vi "getControlData_singleAxis_linear.vi"(11 "system matricec path":path=path "C:/Users/arnold/Documents/MATLAB/AFM_MPC/data/exp_multiAxis.csv") -> (2 "AllMatrix":dbl[](array[numeric]), 3 "ControlParamsMpc":T1={"umax"=3.0, "NS"=0, "ref_f_VEC"=[0.0, 0.0], "Nu11_22"=[0.0, 0.0], "u0"=[0.0, 0.0]})   [LabVIEW 2017]
uses:
  fpga_VIs/fixed-point/typeDefs/FXPControlParams_distEst.ctl
  <vilib>/Utility/file.llb/Read From Spreadsheet File (DBL).vi
panel:
  # "This vi gets control data from a .csv file. It expects the data in\nthe following format:\n| B,   Ki       |\n| L,    Nbar |\n|K',   Ns      |\n|C',   Nd     |\n|Arn,  ref    |\n|.         0      |\n|.         0      |"
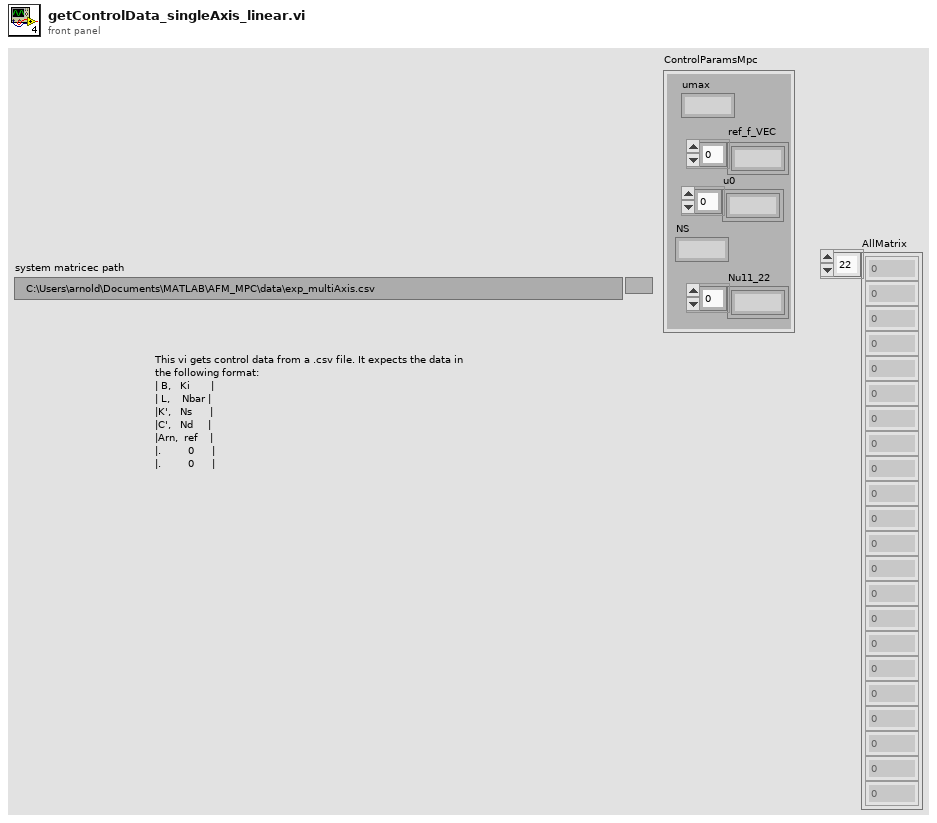
[diagram p1: front panel]
types:
  T1 = typedef "FXPControlParams_distEst.ctl" = cluster{"umax":fxp<+/-,18,5>, "NS":u8, "ref_f_VEC":fxp<+/-,32,5>[], "Nu11_22":fxp<+/-,32,5>[], "u0":fxp<+/-,32,5>[]}
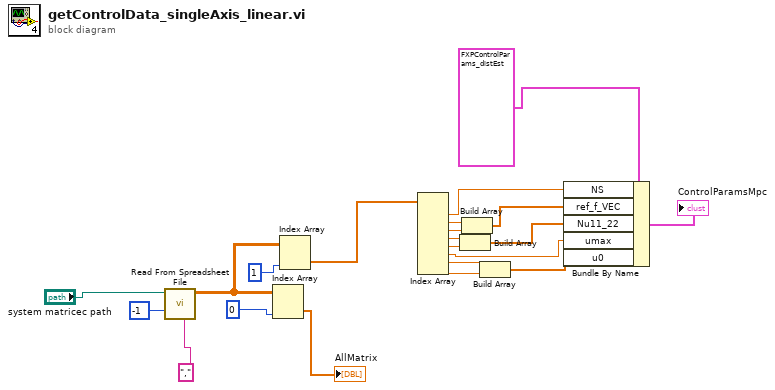
[diagram p0: block diagram]
diagram:
  n1 = call-poly <vilib>:"Read From Spreadsheet File.vi"("delimiter (\\t)"=",", "number of rows (all:-1)"=-1, "file path (dialog if empty)"="system matricec path") -> ("all rows"=w16:dbl[][])  [unwired: 4 in, 4 out]
  n2 = Index Array(array=w16, index (col)=0 ("dimension size")) -> (element=→"AllMatrix":dbl[])  [unwired: 1 in]
  n3 = Index Array(array=w16, index (col)=1 ("dimension size")) -> (element=w19:dbl[])  [unwired: 1 in]
  n4 = Index Array(array=w19) -> (element #1=w20:dbl, element #2=w11:dbl, element #3=w10:dbl, element #4=w8:dbl, element #5=w7:dbl, element #6=w4:dbl, element #7=w3:dbl, element #8=w2:dbl)  [unwired: 8 in]
  n5 = Build Array(w8, w7) -> (w6:dbl[])
  n6 = Build Array(w11, w10) -> (w9:dbl[])
  n7 = Build Array(w3, w2) -> (w1:dbl[])
  n8 = Bundle By Name(cluster=T1 {"umax"=3.0, "NS"=0, "ref_f_VEC"=[0.0, 0.0], "Nu11_22"=[0.0, 0.0], "u0"=[0.0, 0.0]} ("ControlParamsMpc 2"), "NS"=w20, "ref_f_VEC"=w9, "Nu11_22"=w6, "umax"=w4, "u0"=w1) -> (→"ControlParamsMpc":T1)
